vi "Configure Time Interval.vi"(8 "error in (no error)":errorcluster, 10 "Enable Common (Disable)":bool, 11 "VISA resource name":refnum<visa-resource-name>) -> (0 "error out":errorcluster, 3 "VISA resource name out":refnum<visa-resource-name>)   [LabVIEW 2018, in "Counter.lvlib" / "PICOTEST U62XXA series.lvlib"]
doc: "Configure settings required for Time Interval measurement between channels 1 and 2.\n\n<B>Note:</B>\n The U6220A model <B>does not</B> support the \"Time Interval\" commands.\n\n The measurement arming is coupled to Auto with no delay. Arming can be changed by calling any of the Arming VIs. Both channels 1 and 2 have auto-trigger enabled at 50% with a positive slope."
uses:
  PICOTEST U62XXA series.lvlib
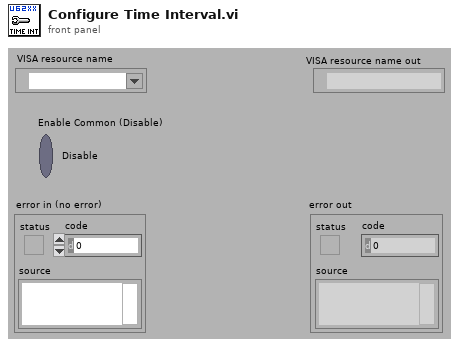
[diagram p1: front panel]
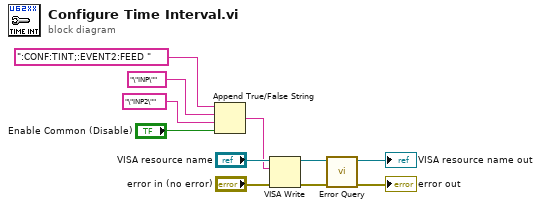
[diagram p0: block diagram]
diagram:
  n1 = Append True/False String(1:"Enable Common (Disable)", 2:"\"INP2\"" ("true string"), 3:"\"INP\"" ("true string"), 4:":CONF:TINT;:EVENT2:FEED " ("string (\"\")")) -> (0:w1:string)
  n2 = VISA Write(VISA resource name="VISA resource name", write buffer=w1, error in (no error)="error in (no error)") -> (VISA resource name out=w5:refnum<visa-resource-name>, error out=w4:errorcluster)  [unwired: 1 out]
  n3 = call "Error Query.vi"("error in (no error)"=w4, "VISA resource name"=w5) -> ("error out"=→"error out":errorcluster, "VISA resource name out"=→"VISA resource name out":refnum<visa-resource-name>)  [unwired: 6 in, 2 out]
